vi "getScanParameters.vi"(8 "error in":T2) -> (0 "error out":T2, 3 "Output Scan Cluster":T1={"Lines"=-2147483648, "Columns"=-2147483648, "X Range "=-inf, "Y Range "=-inf, "Pixel Size"=-inf, "Origin X"=-inf, "Origin Y"=-inf, "Rotation"=-inf, "Sample Time"=-inf} {"Sample Time" format="%#_g µs"; "Rotation" format="%#_g deg"; "Origin Y" format="%#_g nm"; "Origin X" format="%#_g nm"; "Pixel Size" format="%#_g nm"; "Y Range" format="%#_g nm"; "X Range" format="%#_g nm"; "Columns" max=250; "Lines" max=250})   [LabVIEW 2016]
doc: "Retrieves the current values that are set in the scan cluster. For more inforamtion on the parameters that are read out by this VI, please refer to the description of SetScanParameters.vi."
uses:
  Controls/Error_Out.ctl
  Controls/Scan_Parameters.ctl
  Files_ASC500/DLL/ASC500_RemoteControlV27.dll
panel:
  in  "Scan Parameters Cluster":T1={"Lines"=-2147483648, "Columns"=-2147483648, "X Range "=-inf, "Y Range "=-inf, "Pixel Size"=-inf, "Origin X"=-inf, "Origin Y"=-inf, "Rotation"=-inf, "Sample Time"=-inf} {"Sample Time" format="%#_g µs"; "Rotation" format="%#_g deg"; "Origin Y" format="%#_g nm"; "Origin X" format="%#_g nm"; "Pixel Size" format="%#_g nm"; "Y Range" format="%#_g nm"; "X Range" format="%#_g nm"; "Columns" max=250; "Lines" max=250}
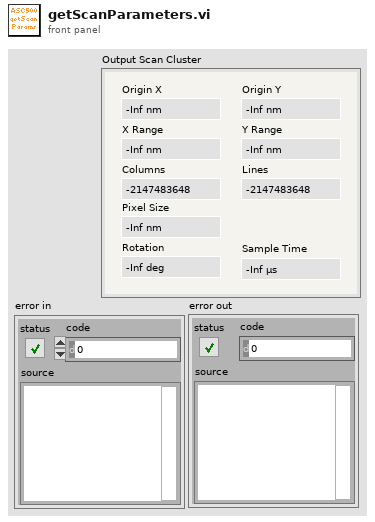
[diagram p1: front panel]
types:
  T1 = typedef "Scan_Parameters.ctl" = cluster{"Lines":i32, "Columns":i32, "X Range ":sgl, "Y Range ":sgl, "Pixel Size":sgl, "Origin X":sgl, "Origin Y":sgl, "Rotation":sgl, "Sample Time":sgl}
  T2 = typedef "Error_Out.ctl" = errorcluster
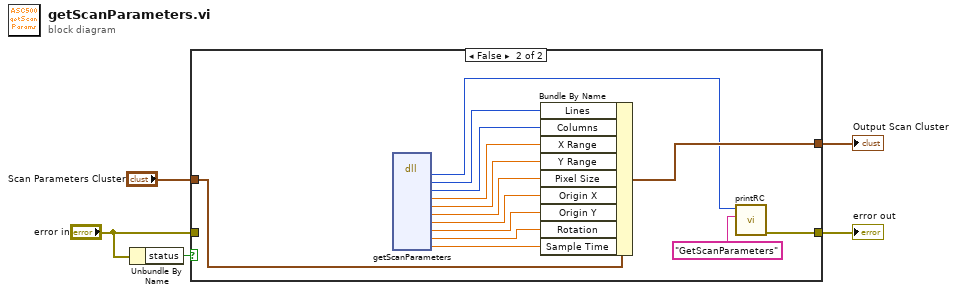
[diagram p0: block diagram]
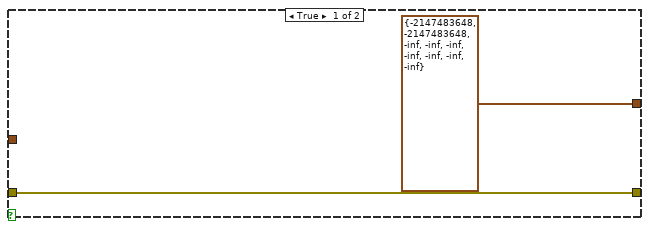
[diagram p2: hidden frame]
diagram:
  n1 = Unbundle By Name("error in") -> ("status"=w4:bool)
  n2 = case shown="False" w4 {
    tunnel: [w6 w19] -> w5
    tunnel: "Scan Parameters Cluster" -> [_ w20]
    tunnel: [T1 {"Lines"=-2147483648, "Columns"=-2147483648, "X Range "=-inf, "Y Range "=-inf, "Pixel Size"=-inf, "Origin X"=-inf, "Origin Y"=-inf, "Rotation"=-inf, "Sample Time"=-inf} ("Scan Parameters Cluster") w21] -> w2
    tunnel: "error in" -> [w6 _]
    frame True {
    }
    frame False {
      n3 = dll-call lib="G:/SCMOperations/Share/ELE/Produkt Information/ASC500/04 Remote Control/02 development versions/2018Nov06/Files_ASC500/DLL/ASC500_RemoteControlV27.dll" fn="getScanParameters"() -> ("Return Code"=w17:i32, "lines"=w16:i32, "columns"=w15:i32, "xRange"=w14:sgl, "yRange"=w13:sgl, "pixelSize"=w12:sgl, "xOffset"=w11:sgl, "yOffset"=w10:sgl, "deg"=w9:sgl, "sampTime"=w8:sgl)  [unwired: 12 in, 2 out]
      n4 = Bundle By Name(cluster=w20, "Lines"=w16, "Columns"=w15, "X Range"=w14, "Y Range"=w13, "Pixel Size"=w12, "Origin X"=w11, "Origin Y"=w10, "Rotation"=w9, "Sample Time"=w8) -> (w21:T1)
      n5 = call "printRC.vi"("additional information"="GetScanParameters", "RC"=w17) -> ("error out"=w19:T2)  [unwired: 9 in]
    }
  }
  "error out" <- w5
  "Output Scan Cluster" <- w2
